vi "AM_OutputSignal.vi"() -> ()   [LabVIEW 2011]
uses:
  <vilib>/sound2/lvsound2.llb/Sound Data Format.ctl
  <vilib>/sound2/lvsound2.llb/Sampling Mode.ctl
  <vilib>/sound2/lvsound2.llb/Sound Output Set Volume (Single).vi
  <vilib>/sound2/lvsound2.llb/Sound Output Write (DBL).vi
panel:
  in  "Signal":waveform(dbl)[](array[waveform])
  in  "Sound Format":T1={"sample rate (S/s)"=22050.0, "number of channels"=2, "bits per sample"=16}
  in  "Number of Samples/Iteration":i32=10000
  in  "Device ID":u32
  in  "stop":bool
  out "Loop Index":i32
  in  "Volume":dbl(slide)=79.59183673469389 scale=0.0..100.0
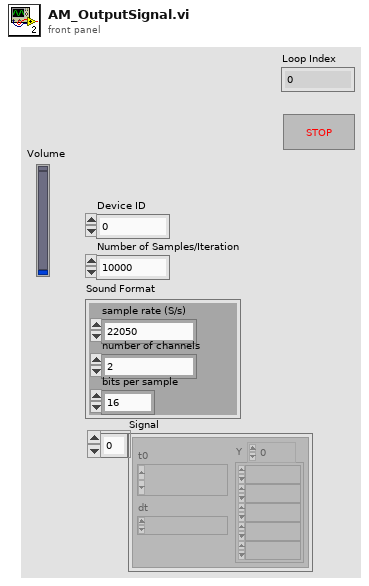
[diagram p1: front panel]
types:
  T1 = typedef "Sound Data Format.ctl" = cluster{"sample rate (S/s)":dbl, "number of channels":i32, "bits per sample":i32}
  T2 = typedef "Sampling Mode.ctl" = i32
  T3 = typedef "Sound Output Task ID.ctl" = u32
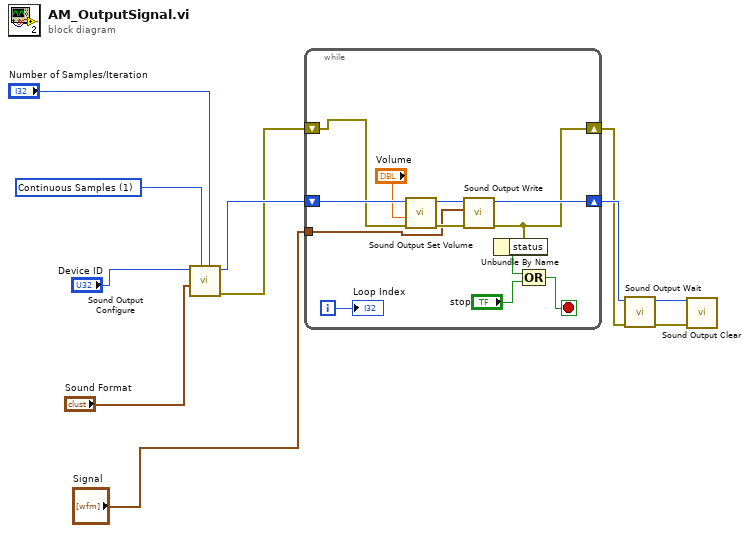
[diagram p0: block diagram]
diagram:
  w8 = T2 1 items=["Finite Samples", "Continuous Samples"] ("sample mode")
  n1 = call <vilib>:"Sound Output Configure.vi"("number of samples/ch"="Number of Samples/Iteration", "sample mode"=w8, "sound format"="Sound Format", "device ID"="Device ID") -> ("error out"=w10:errorcluster, "task ID"=w11:T3)  [unwired: 6 in]
  n2 = while {
    shift-right: [w17] -> w3
    shift-left: w10 -> [w14]
    shift-right: [w23] -> w4
    shift-left: w11 -> [w21]
    tunnel: "Signal" -> [w13]
    i -> [w22]
    stop <- w18 stop-if-true
    n3 = call-poly <vilib>:"Sound Output Set Volume.vi"("error in (no error)"=w14, "volume"="Volume", "task ID"=w21) -> ("error out"=w19:errorcluster, "task ID out"=w20:T3)  [unwired: 7 in]
    n4 = call-poly <vilib>:"Sound Output Write.vi"("error in (no error)"=w19, "data"=w13, "task ID"=w20) -> ("error out"=w17:errorcluster, "task ID out"=w23:T3)  [unwired: 7 in]
    n5 = Unbundle By Name(w17) -> ("status"=w16:bool)
    n6 = Compound Arithmetic op=OR(w16, "stop") -> (w18:bool)
    "Loop Index" <- w22
  }
  n7 = call <vilib>:"Sound Output Wait.vi"("error in (no error)"=w3, "task ID"=w4) -> ("error out"=w5:errorcluster, "task ID out"=w6:T3)  [unwired: 8 in]
  n8 = call <vilib>:"Sound Output Clear.vi"("error in (no error)"=w5, "task ID"=w6) -> ()  [unwired: 9 in, 1 out]
